vi "EXDIR-YAML_Recursive_YAML_Lines_to_Dictionary_ATTEMPT2.vi"(9 "End Index":i32, 10 "Start Index":i32, 11 "ENTIRE Array of YAML Lines":string[](array[string])) -> (1 "items":cluster{"key":variant, "value":variant}[](array[cluster]), 3 "dictionary out":T1)   [LabVIEW 2016]
uses:
  <userlib>/_OpenG.lib/dictionary/dictionary.llb/Dictionary Object RefNum__ogtk.ctl
  <userlib>/_OpenG.lib/dictionary/dictionary.llb/Dictionary Object RefNum - Enum__ogtk.ctl
  <userlib>/_OpenG.lib/dictionary/dictionary.llb/Dictionary Update (by scalar value)__ogtk.vi
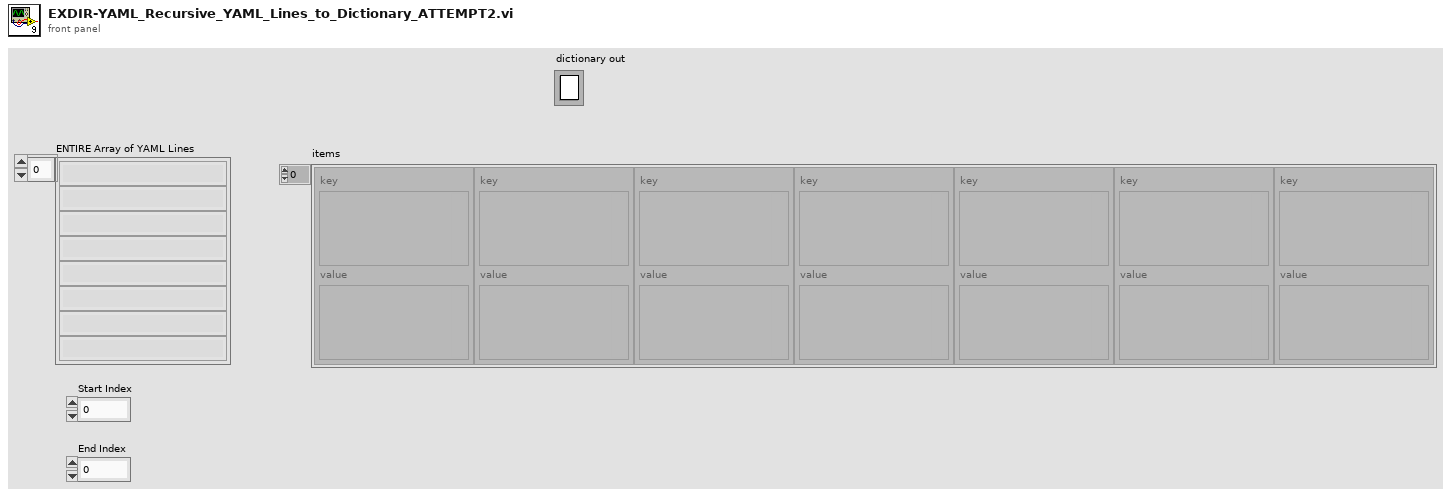
[diagram p1: front panel]
types:
  T1 = typedef "Dictionary Object RefNum__ogtk.ctl" = refnum<k1>
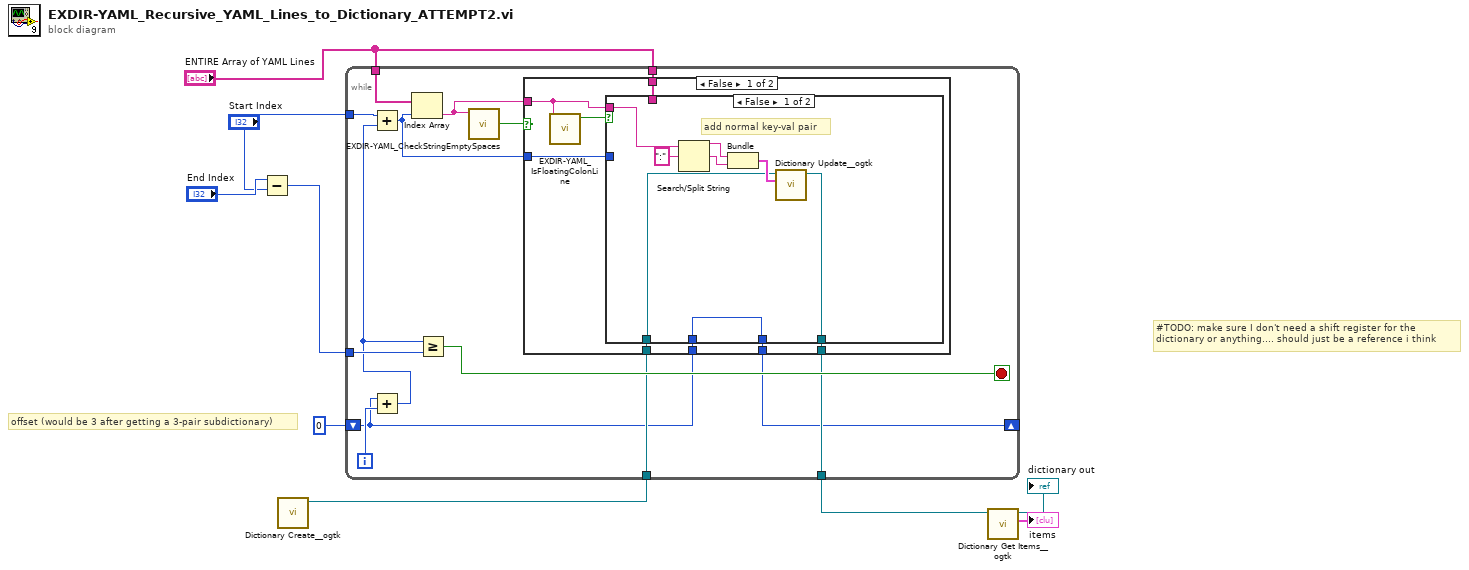
[diagram p0: block diagram]
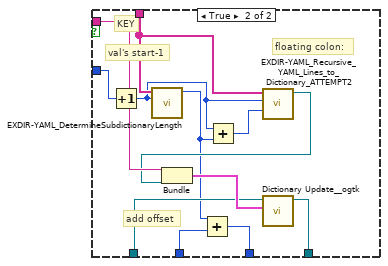
[diagram p2: hidden frame]
diagram:
  # "offset (would be 3 after getting a 3-pair subdictionary)"
  # "#TODO: make sure I don't need a shift register for the\ndictionary or anything.... should just be a reference i think"
  n1 = Subtract(x="End Index", y="Start Index") -> (x-y=w6:i32)
  n2 = call <userlib>:"Dictionary Create__ogtk.vi"() -> ("dictionary out"=w5:T1)  [unwired: 10 in, 1 out]
  n3 = while {
    tunnel: "Start Index" -> [w23]
    tunnel: "ENTIRE Array of YAML Lines" -> [w19]
    tunnel: "ENTIRE Array of YAML Lines" -> [w18]
    tunnel: w6 -> [w17]
    tunnel: w5 -> [w15]
    tunnel: [w14] -> w4
    shift-right: [w10] -> _
    shift-left: 0 -> [w11]
    i -> [w13]
    stop <- w16 stop-if-true
    n4 = Add(x=w11, y=w13) -> (x+y=w12:i32)
    n5 = Add(x=w23, y=w12) -> (x+y=w20:i32)
    n6 = Index Array(array=w18, index=w20) -> (element=w22:string)
    n7 = Greater Or Equal?(x=w12, y=w17) -> (x >= y?=w16:bool)
    n8 = call "EXDIR-YAML_CheckStringEmptySpaces.vi"("String"=w22) -> ("empty or all spaces"=w21:bool)  [unwired: 10 in]
    n9 = case shown="False" w21 {
      tunnel: w22 -> [w30 _]
      tunnel: w20 -> [w29 _]
      tunnel: w19 -> [w28 _]
      tunnel: w15 -> [w27 w53]
      tunnel: [w26 w53] -> w14
      tunnel: w11 -> [w25 w52]
      tunnel: [w24 w52] -> w10
      frame False {
        n10 = call "EXDIR-YAML_IsFloatingColonLine.vi"("Line"=w30) -> ("line ends with floating colon"=w31:bool)  [unwired: 10 in]
        n11 = case shown="False" w31 {
          tunnel: w30 -> [w39 w47]
          tunnel: w29 -> [_ w51]
          tunnel: w28 -> [_ w50]
          tunnel: w27 -> [w34 w44]
          tunnel: [w33 w43] -> w26
          tunnel: w25 -> [w32 w41]
          tunnel: [w32 w40] -> w24
          frame False {
            # "add normal key-val pair"
            n12 = Search/Split String(string=w39, search string/char (-)=":") -> (substring before match=w37:string, match + rest of string=w36:string)  [unwired: 1 in, 1 out]
            n13 = Bundle(w37, w36) -> (w35:cluster{string, string})  [unwired: 1 in]
            n14 = call-poly <userlib>:"Dictionary Update__ogtk.vi"("key-value"=w35, "dictionary"=w34) -> ("dictionary out"=w33:T1)  [unwired: 7 in, 2 out]
          }
          frame True {
            # "add offset"
            # "floating colon:"
            # "val's start-1"
            # "KEY"
            n15 = Increment(x=w51) -> (x+1=w49:i32)
            n16 = call "EXDIR-YAML_DetermineSubdictionaryLength.vi"("start"=w49, "ENTIRE Array of YAML Lines"=w50) -> ("Length"=w42:i32)  [unwired: 8 in, 1 out]
            n17 = Add(x=w42, y=w41) -> (x+y=w40:i32)
            n18 = Add(x=w49, y=w42) -> (x+y=w48:i32)
            n19 = call "EXDIR-YAML_Recursive_YAML_Lines_to_Dictionary_ATTEMPT2.vi"("End Index"=w48, "Start Index"=w49, "ENTIRE Array of YAML Lines"=w50) -> ("dictionary out"=w46:T1)  [unwired: 7 in, 1 out]
            n20 = Bundle(w47, "dictionary out"=w46) -> (w45:cluster{string, "dictionary out":T1})  [unwired: 1 in]
            n21 = call-poly <userlib>:"Dictionary Update__ogtk.vi"("key-value"=w45, "dictionary"=w44) -> ("dictionary out"=w43:T1)  [unwired: 7 in, 2 out]
          }
        }
      }
      frame True {
        # "this line is empty, move along"
      }
    }
  }
  n22 = call <userlib>:"Dictionary Get Items__ogtk.vi"("dictionary"=w4) -> ("items"=→"items":cluster{"key":variant, "value":variant}[], "dictionary out"=→"dictionary out":T1)  [unwired: 8 in, 1 out]
